vi "ReCalc_V2.00.vi"(3 "Berechnen":bool, 4 "Datenspeicher":T2={"Fahrzeugdaten"="", "date/time string"="", "Rolle [Inkr/U]"=0, "Rollenumfang [m]"=0.0, "Rollenträgheit [kgm²]"=0.0, "Zündung [Imp/U]"=0.0, "Getriebe [1:]"=0.0, "Reifenumfang [m] "=0.0, "element"=0.0, "Gl. Mittelwert"=0, "Differenzenquotient"=0, "Polynom"=0, "dT [s]"=0.0, "element"=0.0, "Lufttemperatur [°C]"=0.0, "Luftfeuchtigkeit [%]"=0.0, "Luftdruck [mbar]"=0.0, [], [], "Best Polynomial Fit"=[], [], "Übersetzung ermitteln aus"=0, "[s]"=0.0, "nmin [1/min]"=0.0, "nmax [1/min]"=0.0, "n vom Gas [1/min]"=0.0, "dT ungefiltert [s]"=[], [], "Boolesch"=FALSE, "Serielle Schnittstelle"="COM4", "nKuWe/nRolle 2"=10.0, "v vom Gas [km/h]"=5000.0}) -> ()   [LabVIEW 2014]
uses:
  <vilib>/Utility/miscctls.llb/LVPointTypeDef.ctl
  <vilib>/Analysis/3filter.llb/IIR Filter (DBL).vi
  <vilib>/Analysis/NI_AALBase.lvlib
panel:
  in  "v vom Gas [km/h]":dbl=5000.0
  in  "Legende":bool=TRUE
  out "Fahrzeugdaten":string
  out "Überlagerung":bool
  in  "Überlagern":bool
  out "Übersetzung ermitteln aus":T1(ring)
  in  "Speichern":bool
  out "Reifenumfang [m]":dbl=1.222
  out "Getriebe [1:]":dbl=5.343
  out "Zündung [Imp/U]":dbl=1.0
  out "Rollengeber [Inkr/U]":u16=200
  out "Luftdruck [mbar]":dbl=1013.0
  out "Luftfeuchtigkeit [%]":dbl=50.0
  out "Lufttemperatur [°C]":dbl=20.0
  in  "Stopp":bool
  in  "Rollenträgheit [kgm²]":dbl=0.402
  in  "Gl. Mittelwert":u8=35
  in  "Differenzenquotient":u8=12
  in  "n vom Gas [1/min]":dbl=5000.0
  out "Rollenumfang [m]":dbl=0.613 format="%.3f"
  out "Datum, Zeit":string
  out "Untersetzung aus:":dbl=2.68 format="%.2f"
  in  "Drucken":bool
  out "Pmax":string
  out "Ergebnis":string
  out "XY-Graph":cluster{dbl[], dbl[]}[](graph)
  in  "Öffnen":bool
  out "korr":dbl
  out "[s]":dbl=5.0
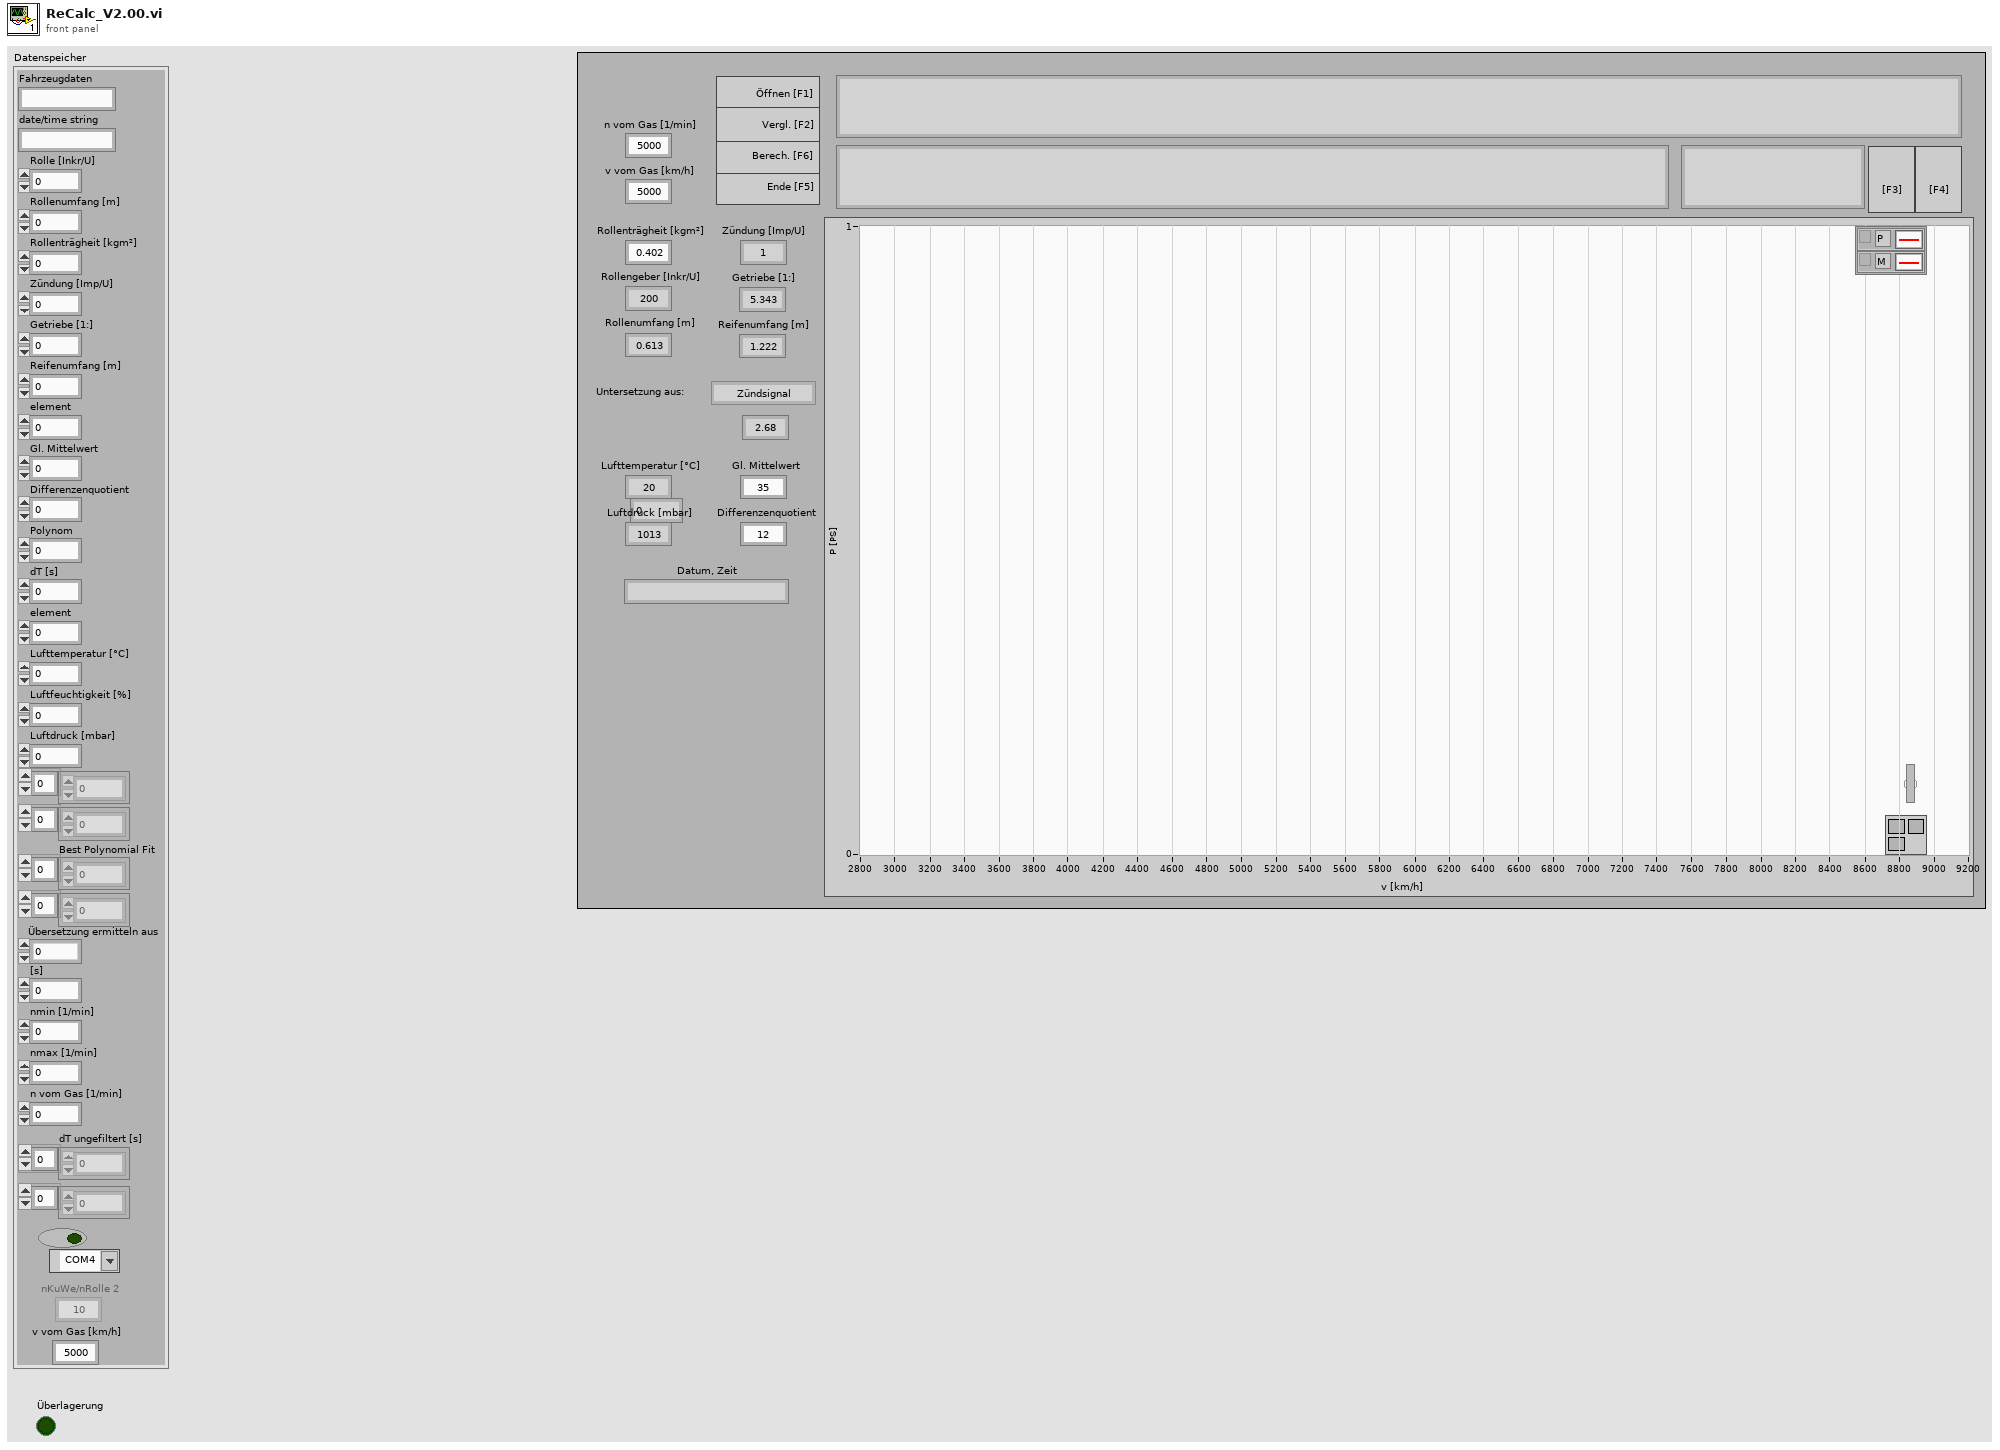
[diagram p1: front panel]
types:
  T1 = enum8{"Zündsignal", "Getriebe & Reifen", "nKuWe / nRolle", "Vario [km/h]"}
  T2 = cluster{"Fahrzeugdaten":string, "date/time string":string, "Rolle [Inkr/U]":u16, "Rollenumfang [m]":dbl, "Rollenträgheit [kgm²]":dbl, "Zündung [Imp/U]":dbl, "Getriebe [1:]":dbl, "Reifenumfang [m] ":dbl, "element":dbl, "Gl. Mittelwert":u8, "Differenzenquotient":u8, "Polynom":u8, "dT [s]":dbl, "element":dbl, "Lufttemperatur [°C]":dbl, "Luftfeuchtigkeit [%]":dbl, "Luftdruck [mbar]":dbl, dbl[], dbl[], "Best Polynomial Fit":dbl[], dbl[], "Übersetzung ermitteln aus":u8, "[s]":dbl, "nmin [1/min]":dbl, "nmax [1/min]":dbl, "n vom Gas [1/min]":dbl, "dT ungefiltert [s]":dbl[], i32[], "Boolesch":bool, "Serielle Schnittstelle":refnum<visa-resource-name>, "nKuWe/nRolle 2":dbl, "v vom Gas [km/h]":dbl}
  T3 = typedef "LVPointTypeDef.ctl" = cluster{"Horizontal":i16, "Vertical":i16}
  T4 = enum16{"Zündsignal", "Getriebe & Reifen", "nKuWe / nRolle", "Vario (km/h)"}
  T5 = cluster{"Fahrzeugdaten":string, "date/time string":string, "Rolle [Inkr/U]":u16, "Rollenumfang [m]":dbl, "Rollenträgheit [kgm²]":dbl, "Zündung [Imp/U]":dbl, "Getriebe [1:]":dbl, "Reifenumfang [m] ":dbl, "element":dbl, "Gl. Mittelwert":u8, "Differenzenquotient":u8, "Polynom":u8, "dT [s]":dbl, "element":dbl, "Lufttemperatur [°C]":dbl, "Luftfeuchtigkeit [%]":dbl, "Luftdruck [mbar]":dbl, dbl[], dbl[], "Best Polynomial Fit":dbl[], dbl[], "Übersetzung ermitteln aus":u8, "[s]":dbl, "nmin [1/min]":dbl, "nmax [1/min]":dbl, "n vom Gas [1/min]":dbl, "dT-Array [s]":dbl[], i32[], "Boolesch":bool, "Serielle Schnittstelle":refnum<visa-resource-name>, "nKuWe/nRolle":dbl, "v vom Gas [km/h]":dbl}
  T6 = enum8{"Enabled", "Disabled", "Disabled and Grayed Out"}
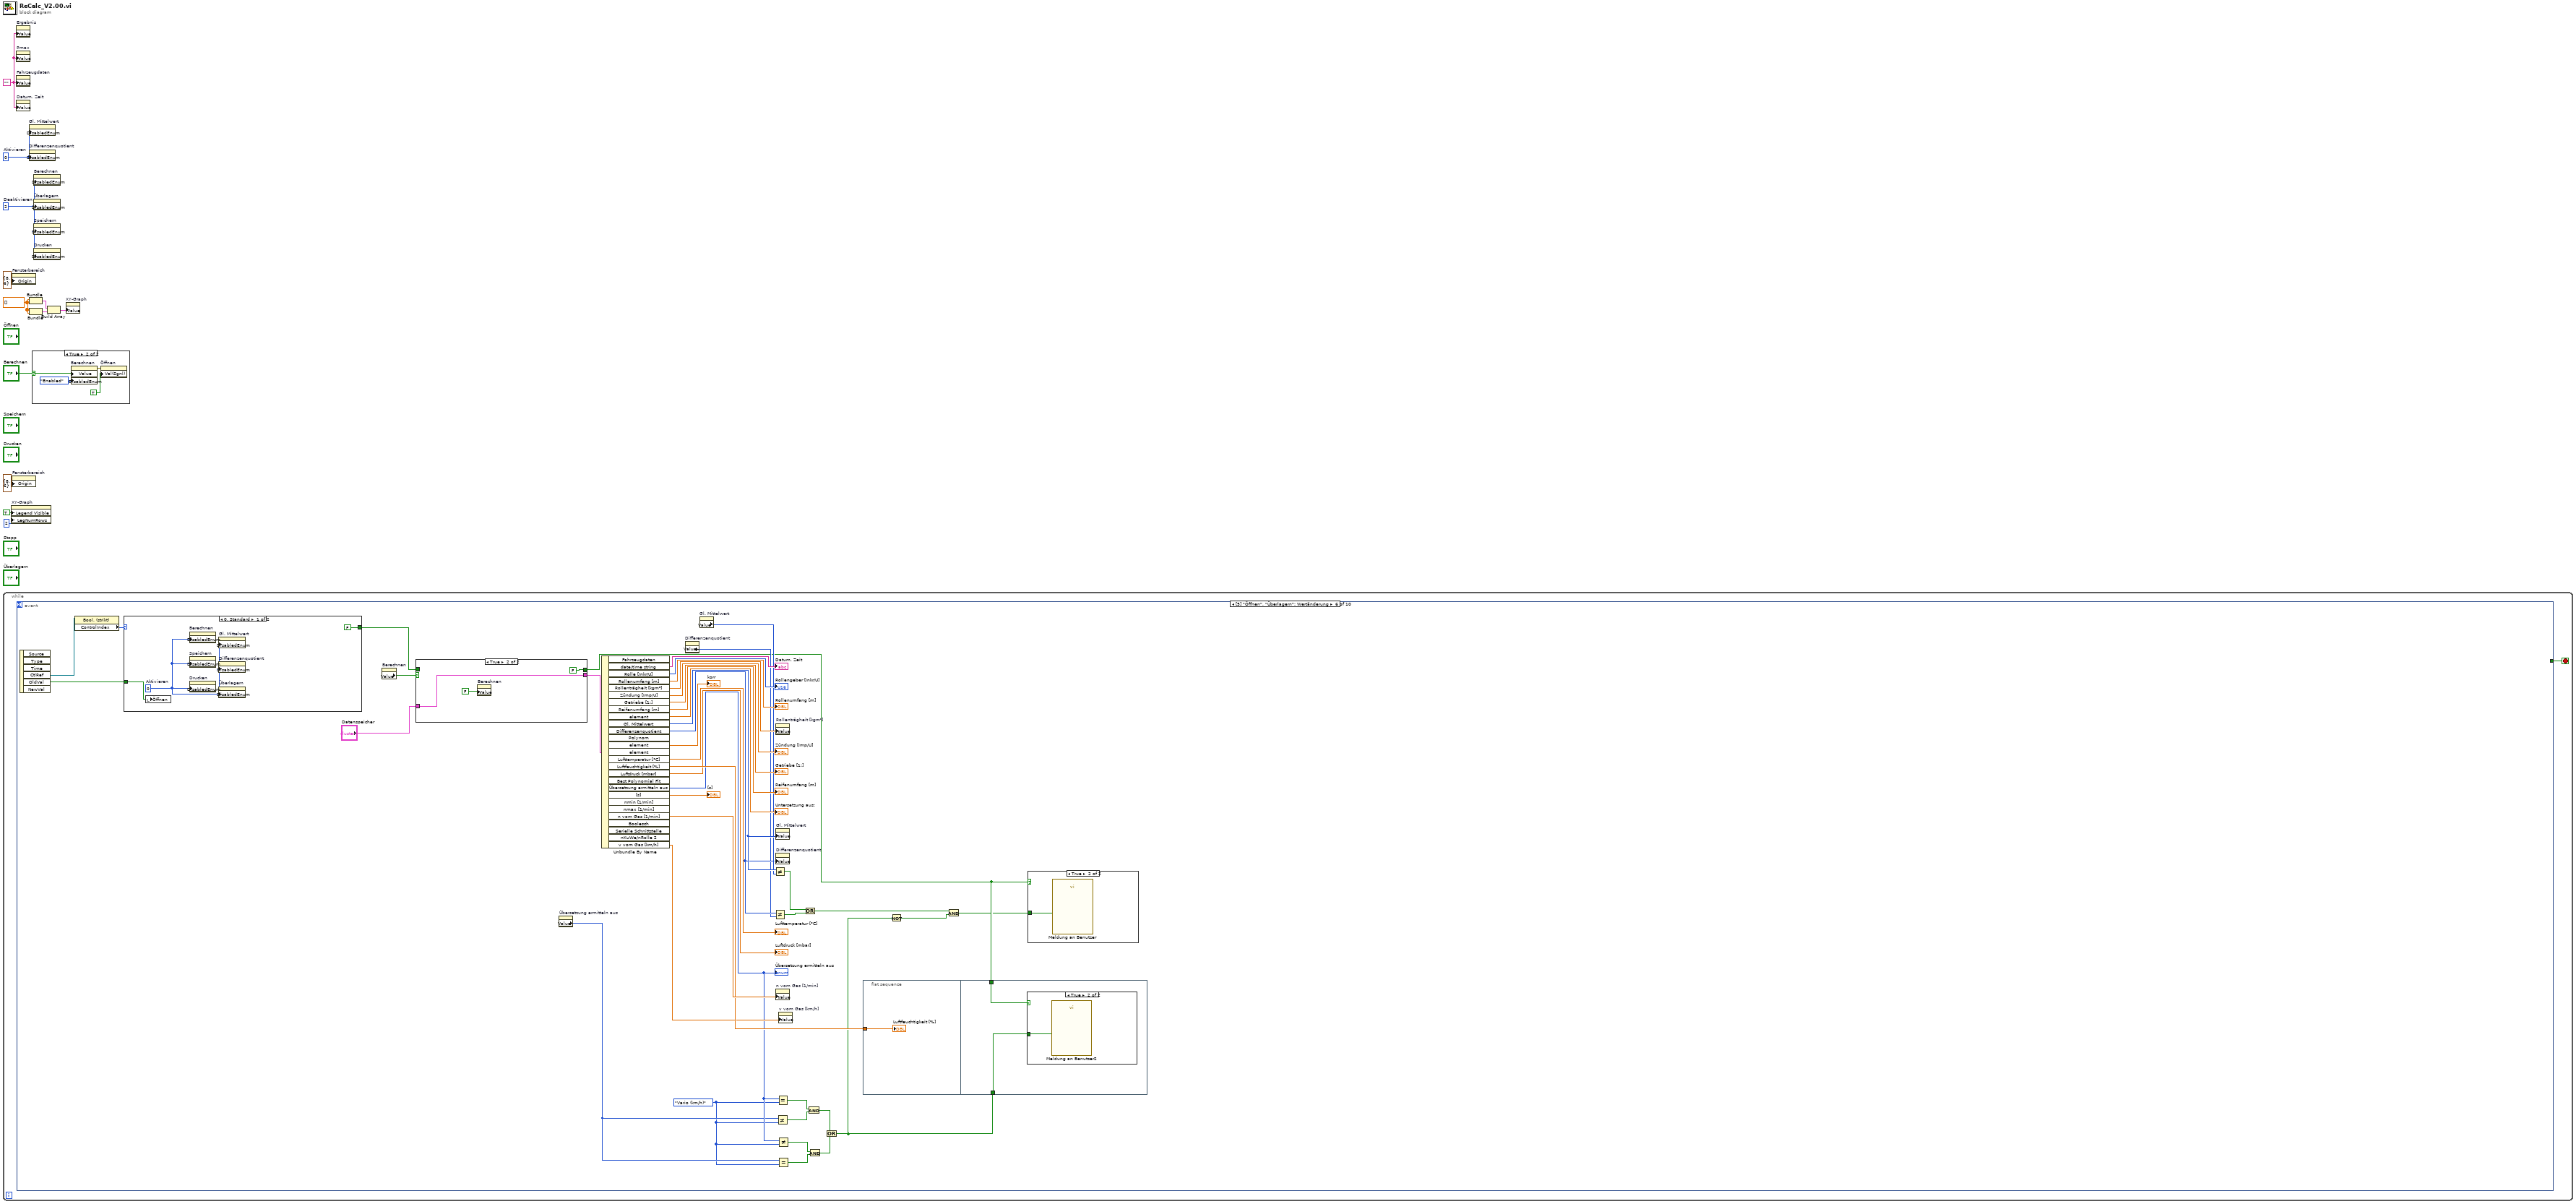
[diagram p0: block diagram]
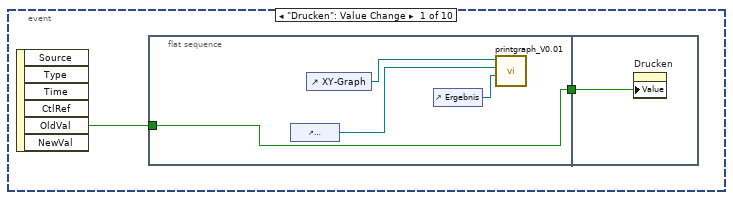
[diagram p3: hidden frame]
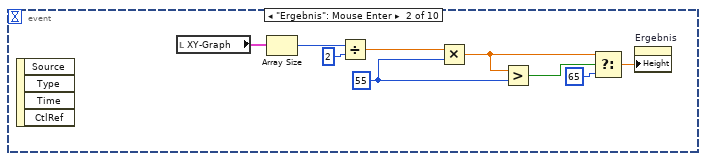
[diagram p4: hidden frame]
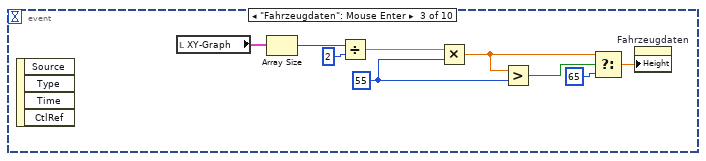
[diagram p5: hidden frame]
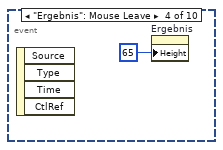
[diagram p6: hidden frame]
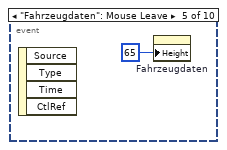
[diagram p7: hidden frame]
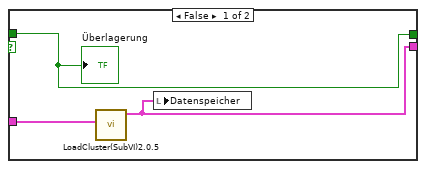
[diagram p9: hidden frame]
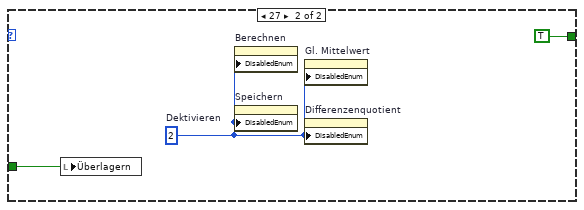
[diagram p11: hidden frame]
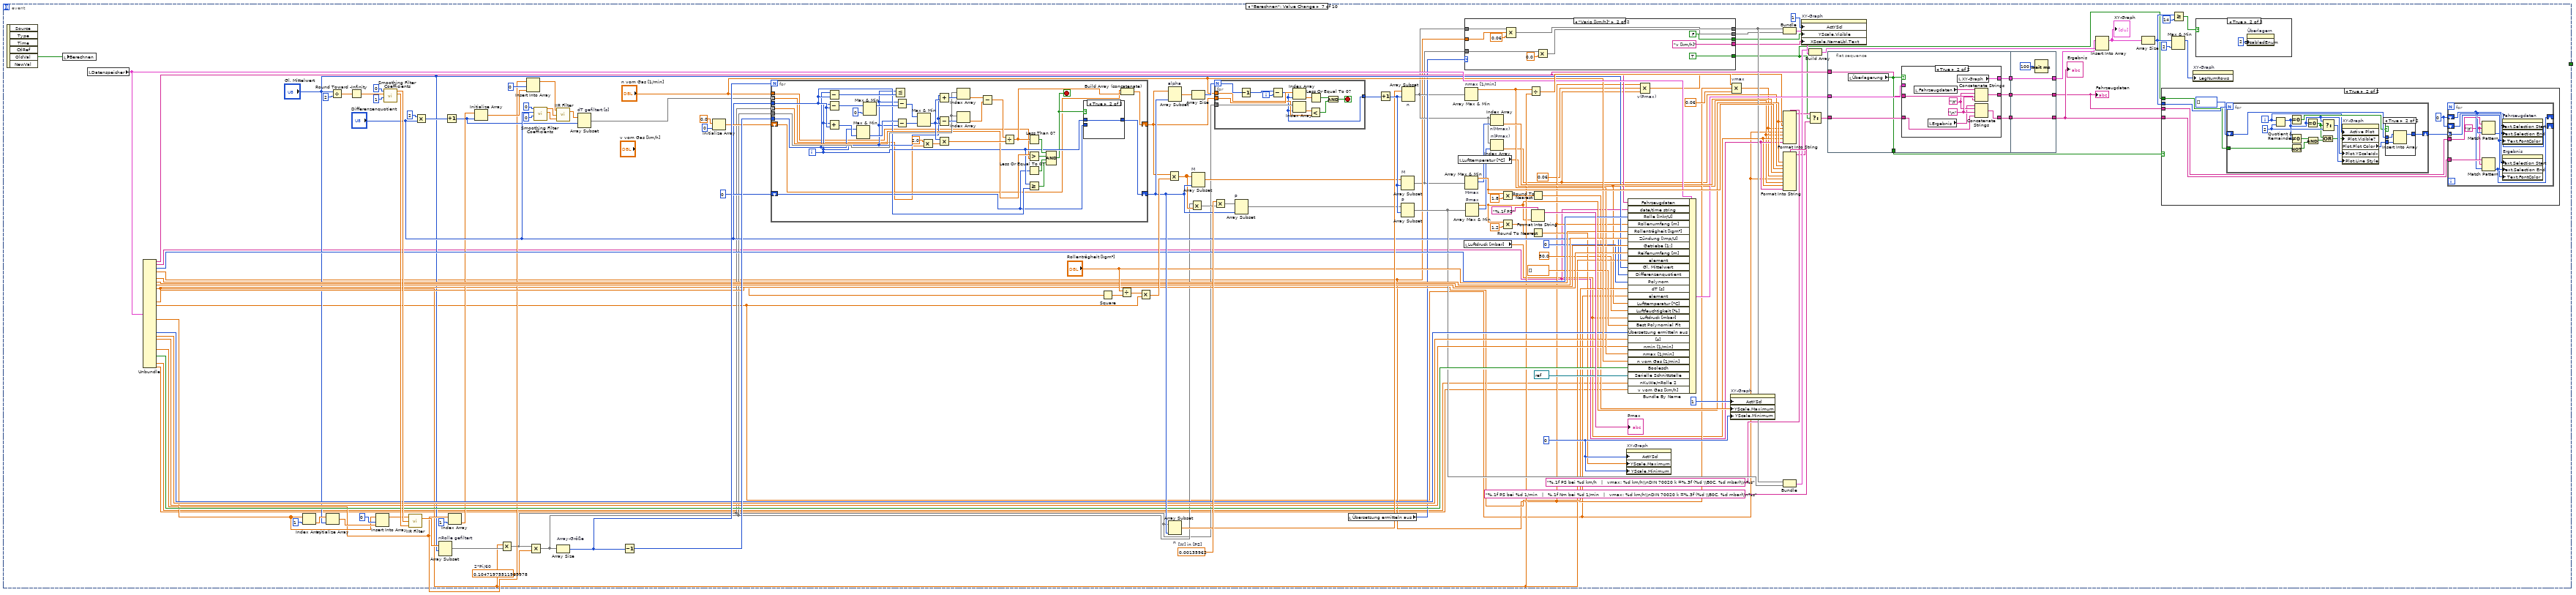
[diagram p12: hidden frame]
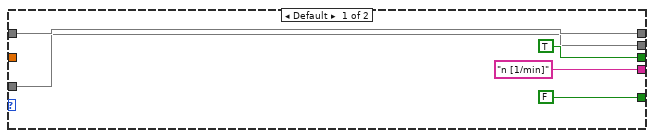
[diagram p13: hidden frame]
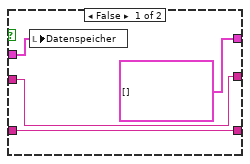
[diagram p15: hidden frame]
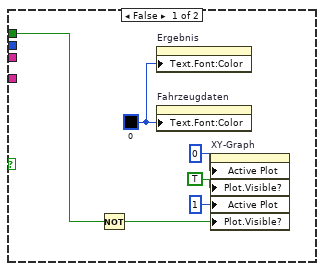
[diagram p16: hidden frame]
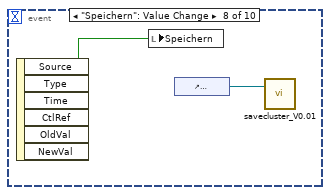
[diagram p19: hidden frame]
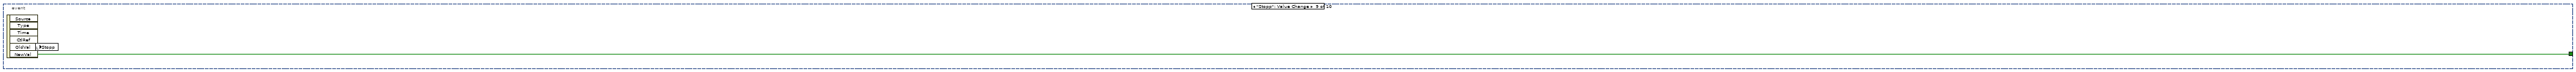
[diagram p20: hidden frame]
diagram:
  w2 = 0  # Aktivieren
  w8 = dbl[] []
  w4 = 2  # Deaktivieren
  w12 = ""
  n1 = while {
    stop <- w13 stop-if-true
    n2 = event shown="[5] \"Öffnen\", \"Überlagern\": Wertänderung" {
      selector: _ -> [_ _ _ _ _ _ _ _ _ _]
      dyn-events: _ -> [_ _ _ _ _ _ _ _ _ _]
      timeout: _ -> [_ _ _ _ _ _ _ _ _ _]
      tunnel: [_ _ _ _ _ _ _ _ w367 _] -> w13
      event "Drucken": Value Change {
        n3 = event-data() -> ("OldVal"=w15:bool)  [unwired: 1 in, 5 out]
        n4 = flat-sequence {
          tunnel: w15 -> [w19]
          tunnel: [w19] -> w14
          tunnel: w14 -> [w20]
          frame #0 {
            n5 = control-ref of="Fahrzeugdaten"() -> (w17:refnum<vi>)
            n6 = control-ref of="XY-Graph"() -> (w18:refnum<vi>)
            n7 = control-ref of="Ergebnis"() -> (w16:refnum<vi>)
            n8 = call "printgraph_V0.01.vi"("reference 2"=w16, "Fahrzeugdaten"=w17, "XYGraph (Eingang)"=w18) -> ()  [unwired: 9 in]
          }
          frame #1 {
            n9 = property on="Drucken" class="Bool. (strikt)"("Value"=w20) -> ()  [unwired: 2 in, 2 out]
          }
        }
      }
      event "Ergebnis": Mouse Enter {
        w23 = u32 55 ("Größe:Höhe")
        n10 = event-data() -> ()  [unwired: 1 in, 4 out]
        n11 = local read "XY-Graph"() -> (w29:cluster{dbl[], dbl[]}[])
        n12 = Array Size(array=w29) -> (size(s)=w28:i32)
        n13 = Divide(x=w28, y=2) -> (x/y=w26:dbl)
        n14 = Multiply(x=w26, y=w23) -> (x*y=w24:dbl)
        n15 = Greater?(x=w24, y=w23) -> (0:w25:bool)
        n16 = Select(t=w24, s=w25, f=u32 65 ("Größe:Höhe")) -> (s? t:f=w22:dbl)
        n17 = property on="Ergebnis" class="Str"("Height"=w22) -> ()  [unwired: 2 in, 2 out]
      }
      event "Fahrzeugdaten": Mouse Enter {
        w32 = u32 55 ("Größe:Höhe")
        n18 = event-data() -> ()  [unwired: 1 in, 4 out]
        n19 = local read "XY-Graph"() -> (w38:cluster{dbl[], dbl[]}[])
        n20 = Array Size(array=w38) -> (size(s)=w37:i32)
        n21 = Divide(x=w37, y=2) -> (x/y=w35:dbl)
        n22 = Multiply(x=w35, y=w32) -> (x*y=w33:dbl)
        n23 = Greater?(x=w33, y=w32) -> (0:w34:bool)
        n24 = Select(t=w33, s=w34, f=u32 65 ("Größe:Höhe")) -> (s? t:f=w31:dbl)
        n25 = property on="Fahrzeugdaten" class="Str"("Height"=w31) -> ()  [unwired: 2 in, 2 out]
      }
      event "Ergebnis": Mouse Leave {
        n26 = event-data() -> ()  [unwired: 1 in, 4 out]
        n27 = property on="Ergebnis" class="Str"("Height"=u32 65 ("Größe:Höhe")) -> ()  [unwired: 2 in, 2 out]
      }
      event "Fahrzeugdaten": Mouse Leave {
        n28 = event-data() -> ()  [unwired: 1 in, 4 out]
        n29 = property on="Fahrzeugdaten" class="Str"("Height"=u32 65 ("Größe:Höhe")) -> ()  [unwired: 2 in, 2 out]
      }
      event "Öffnen", "Überlagern": Value Change {
        w50 = T4."Vario (km/h)"
        n30 = event-data() -> ("CtlRef"=w81:refnum<vi>, "OldVal"=w79:bool)  [unwired: 1 in, 4 out]
        n31 = property class="Bool. (strikt)"(reference=w81) -> ("ControlIndex"=w80:i32)  [unwired: 1 in, 2 out]
        n32 = case shown="0, Standard" w80 {
          tunnel: w79 -> [w96 w99]
          tunnel: [FALSE ("Überlagerung") TRUE ("Überlagerung")] -> w78
          frame 0, Default {
            w94 = 0  # Aktivieren
            n33 = local write "Öffnen"(w96) -> ()
            n34 = property on="Berechnen" class="Bool. (strikt)"("DisabledEnum"=w94) -> ()  [unwired: 2 in, 2 out]
            n35 = property on="Speichern" class="Bool. (strikt)"("DisabledEnum"=w94) -> ()  [unwired: 2 in, 2 out]
            n36 = property on="Drucken" class="Bool. (strikt)"("DisabledEnum"=w94) -> ()  [unwired: 2 in, 2 out]
            n37 = property on="Gl. Mittelwert" class="DigWert (strikt)"("DisabledEnum"=w94) -> ()  [unwired: 2 in, 2 out]
            n38 = property on="Differenzenquotient" class="DigWert (strikt)"("DisabledEnum"=w94) -> ()  [unwired: 2 in, 2 out]
            n39 = property on="Überlagern" class="Bool. (strikt)"("DisabledEnum"=w94) -> ()  [unwired: 2 in, 2 out]
          }
          frame 27 {
            w97 = 2  # Dektivieren
            n40 = local write "Überlagern"(w99) -> ()
            n41 = property on="Berechnen" class="Bool. (strikt)"("DisabledEnum"=w97) -> ()  [unwired: 2 in, 2 out]
            n42 = property on="Speichern" class="Bool. (strikt)"("DisabledEnum"=w97) -> ()  [unwired: 2 in, 2 out]
            n43 = property on="Gl. Mittelwert" class="DigWert (strikt)"("DisabledEnum"=w97) -> ()  [unwired: 2 in, 2 out]
            n44 = property on="Differenzenquotient" class="DigWert (strikt)"("DisabledEnum"=w97) -> ()  [unwired: 2 in, 2 out]
          }
        }
        n45 = property on="Berechnen" class="Bool. (strikt)"() -> ("Value"=w63:bool)  [unwired: 2 in, 2 out]
        n46 = case shown="True" w63 {
          tunnel: "Datenspeicher" -> [w85 w88]
          tunnel: w78 -> [w86 _]
          tunnel: [w84 w88] -> w64
          tunnel: [w86 FALSE] -> w45
          frame False {
            n47 = call "LoadCluster(SubVI)2.0.5.vi"("Datenspeicher"=w85) -> ("Value"=w84:T5)  [unwired: 10 in]
            n48 = local write "Datenspeicher"(w84) -> ()
            "Überlagerung" <- w86
          }
          frame True {
            n49 = property on="Berechnen" class="Bool. (strikt)"("Value"=FALSE) -> ()  [unwired: 2 in, 2 out]
          }
        }
        n50 = property on="Übersetzung ermitteln aus" class="Enum (strikt)"() -> ("Value"=w51:T1)  [unwired: 2 in, 2 out]
        n51 = Unbundle By Name(w64) -> ("date/time string"=→"Datum, Zeit":string, "Rolle [Inkr/U]"=→"Rollengeber [Inkr/U]":u16, "Rollenumfang [m]"=→"Rollenumfang [m]":dbl, "Rollenträgheit [kgm²]"=w68:dbl, "Zündung [Imp/U]"=→"Zündung [Imp/U]":dbl, "Getriebe [1:]"=→"Getriebe [1:]":dbl, "Reifenumfang [m]"=→"Reifenumfang [m]":dbl, "element"=→"Untersetzung aus:":dbl, "Gl. Mittelwert"=w62:u8, "Differenzenquotient"=w60:u8, "element"=→"korr":dbl, "Lufttemperatur [°C]"=→"Lufttemperatur [°C]":dbl, "Luftfeuchtigkeit [%]"=w75:dbl, "Luftdruck [mbar]"=→"Luftdruck [mbar]":dbl, "Übersetzung ermitteln aus"=w52:u8, "[s]"=→"[s]":dbl, "n vom Gas [1/min]"=w77:dbl, "v vom Gas [km/h]"=w55:dbl)  [unwired: 9 out]
        "Übersetzung ermitteln aus" <- w52
        n52 = property on="Differenzenquotient" class="DigWert (strikt)"() -> ("Value"=w59:u8)  [unwired: 2 in, 2 out]
        n53 = property on="Gl. Mittelwert" class="DigWert (strikt)"() -> ("Value"=w61:u8)  [unwired: 2 in, 2 out]
        n54 = Not Equal?(x=w62, y=w61) -> (x != y?=w58:bool)
        n55 = Not Equal?(x=w60, y=w59) -> (x != y?=w57:bool)
        n56 = property on="Rollenträgheit [kgm²]" class="DigWert (strikt)"("Value"=w68) -> ()  [unwired: 2 in, 2 out]
        n57 = property on="Gl. Mittelwert" class="DigWert (strikt)"("Value"=w62) -> ()  [unwired: 2 in, 2 out]
        n58 = property on="Differenzenquotient" class="DigWert (strikt)"("Value"=w60) -> ()  [unwired: 2 in, 2 out]
        n59 = property on="n vom Gas [1/min]" class="DigWert (strikt)"("Value"=w77) -> ()  [unwired: 2 in, 2 out]
        n60 = Not Equal?(x=w51, y=w50) -> (x != y?=w53:bool)
        n61 = Equal?(x=w52, y=w50) -> (x = y?=w54:bool)
        n62 = Not Equal?(x=w52, y=w50) -> (x != y?=w49:bool)
        n63 = Equal?(x=w51, y=w50) -> (x = y?=w48:bool)
        n64 = property on="v vom Gas [km/h]" class="DigWert (strikt)"("Value"=w55) -> ()  [unwired: 2 in, 2 out]
        n65 = Or(x=w58, y=w57) -> (x .or. y?=w41:bool)
        n66 = And(x=w54, y=w53) -> (x .and. y?=w47:bool)
        n67 = And(x=w49, y=w48) -> (x .and. y?=w46:bool)
        n68 = Or(x=w47, y=w46) -> (x .or. y?=w43:bool)
        n69 = flat-sequence {
          tunnel: w75 -> [w90]
          tunnel: w45 -> [w92]
          tunnel: w43 -> [w91]
          frame #0 {
            "Luftfeuchtigkeit [%]" <- w90
          }
          frame #1 {
            n70 = case shown="True" w92 {
              tunnel: w91 -> [_ w93]
              frame False {
              }
              frame True {
                n71 = call "Meldung an Benutzer2"("Enable"=w93) -> ()  [unwired: 9 in, 2 out]
              }
            }
          }
        }
        n72 = Not(x=w43) -> (.not. x?=w42:bool)
        n73 = And(x=w41, y=w42) -> (x .and. y?=w44:bool)
        n74 = case shown="True" w45 {
          tunnel: w44 -> [_ w83]
          frame False {
          }
          frame True {
            n75 = call "Meldung an Benutzer"("Enable"=w83) -> ()  [unwired: 9 in, 2 out]
          }
        }
      }
      event "Berechnen": Value Change {
        w210 = 0
        w224 = 0.00135962  # [W] in [PS]
        w231 = 0.10471975511965978  # 2*Pi/60
        n76 = event-data() -> ("OldVal"=w180:bool)  [unwired: 1 in, 5 out]
        n77 = local write "Berechnen"(w180) -> ()
        n78 = local read "Datenspeicher"() -> (w193:T2)
        n79 = Unbundle(w193) -> ("Fahrzeugdaten"=w172:string, "date/time string"=w115:string, "Rolle [Inkr/U]"=w192:u16, "Rollenumfang [m]"=w118:dbl, "Zündung [Imp/U]"=w186:dbl, "Getriebe [1:]"=w185:dbl, "Reifenumfang [m]"=w184:dbl, "element"=w134:dbl, "dT [s]"=w144:dbl, "element"=w112:dbl, w143:dbl[], "Übersetzung ermitteln aus"=w187:u8, "[s]"=w181:dbl, "nmin [1/min]"=w182:dbl, "dT ungefiltert [s]"=w142:dbl[], "Boolesch"=w189:bool, "nKuWe/nRolle 2"=w100:dbl, "v vom Gas [km/h]"=w101:dbl)  [unwired: 14 out]
        n80 = Index Array(array=w143, index=1) -> (element=w198:dbl)
        n81 = Initialize Array(w198, "Gl. Mittelwert") -> (w199:dbl[])
        n82 = Divide(x="Gl. Mittelwert", y=2) -> (x/y=w234:dbl)
        n83 = Round Toward -Infinity(1:w234) -> (0:w233:dbl)
        n84 = Insert Into Array ("In Array einfügen")(array=w143, index=0, new element=w199) -> (w196:dbl[])
        n85 = call <vilib>:"Smoothing Filter Coefficients.vi"("shape"=1, "half-width"=w233, "type"=0) -> ("forward coefficients"=w200:dbl[], "reverse coefficients"=w201:dbl[])  [unwired: 6 in, 1 out]
        n86 = call-poly <vilib>:"IIR Filter.vi"("Forward Coefficients"=w200, "Reverse Coefficients"=w201, "X"=w196) -> ("Filtered X"=w195:dbl[])  [unwired: 1 in, 1 out]
        n87 = Multiply(x=2, y="Differenzenquotient") -> (x*y=w152:i32)
        n88 = Array Subset "nRolle gefiltert"(array=w195, index="Gl. Mittelwert") -> (w136:dbl[])  [unwired: 1 in]
        n89 = Increment(x=w152) -> (x+1=w145:i32)
        n90 = Index Array(array=w142, index=1 ("Index")) -> (element=w150:dbl)
        n91 = Initialize Array(w150, w145) -> (w148:dbl[])
        n92 = Multiply(x=w134, y=w136) -> (x*y=w135:dbl[])
        n93 = Insert Into Array(array=w142, index=0 ("Index"), new element=w148) -> (w147:dbl[])
        n94 = Multiply(x=w135, y=w231) -> (x*y=w138:dbl[])
        n95 = call <vilib>:"Smoothing Filter Coefficients.vi"("shape"=0, "half-width"="Differenzenquotient", "type"=0) -> ("forward coefficients"=w155:dbl[], "reverse coefficients"=w156:dbl[])  [unwired: 6 in, 1 out]
        n96 = call-poly <vilib>:"IIR Filter.vi"("Forward Coefficients"=w155, "Reverse Coefficients"=w156, "X"=w147) -> ("Filtered X"=w146:dbl[])  [unwired: 1 in, 1 out]
        n97 = Array Size "Array-Größe"(array=w138) -> (size(s)=w229:i32)
        n98 = Array Subset "dT gefiltert [s]"(array=w146, index=w145) -> (w137:dbl[])  [unwired: 1 in]
        n99 = Decrement(x=w229) -> (x-1=w230:i32)
        n100 = Initialize Array(0.0 ("y"), 0) -> (w226:dbl[])
        n101 = for {
          N: w229 -> [_]
          tunnel: "Differenzenquotient" -> [w342]
          tunnel: w138 -> [w348]
          tunnel: w230 -> [w341]
          shift-right: [w346] -> w139
          shift-left: w226 -> [w329]
          tunnel: w135 -> [w344] mode=indexing
          tunnel: "n vom Gas [1/min]" -> [w333]
          shift-right: [w332] -> w217
          shift-left: 0 -> [w335]
          tunnel: w137 -> [w328] mode=indexing
          i -> [w336]
          stop <- w334 stop-if-true
          n102 = Subtract(x=w341, y=w342) -> (x-y=w343:i32)
          n103 = Subtract(x=w336, y=w342) -> (x-y=w361:i32)
          n104 = Add(x=w336, y=w342) -> (x+y=w355:i32)
          n105 = Max & Min(x=w341, y=w355) -> (min(x,y)=w356:i32)  [unwired: 1 out]
          n106 = Max & Min(x=w361, y=0) -> (max(x,y)=w359:i32)  [unwired: 1 out]
          n107 = Less Or Equal?(x=w336, y=w343) -> ()  [unwired: 1 out]
          n108 = Subtract(x=w336, y=w359) -> (x-y=w358:i32)
          n109 = Subtract(x=w356, y=w336) -> (x-y=w357:i32)
          n110 = Max & Min(x=w358, y=w357) -> (min(x,y)=w349:i32)  [unwired: 1 out]
          n111 = Multiply(x=2.0, y=w328) -> (x*y=w330:dbl)
          n112 = Add(x=w336, y=w349) -> (x+y=w354:i32)
          n113 = Subtract(x=w336, y=w349) -> (x-y=w353:i32)
          n114 = Multiply(x=w349, y=w330) -> (x*y=w347:dbl)
          n115 = Index Array(array=w348, index=w354) -> (element=w351:dbl)
          n116 = Index Array(array=w348, index=w353) -> (element=w352:dbl)
          n117 = Subtract(x=w351, y=w352) -> (x-y=w350:dbl)
          n118 = Divide(x=w350, y=w347) -> (x/y=w340:dbl)
          n119 = Less Than 0?(x=w340) -> (x < 0?=w338:bool)
          n120 = Greater?(x=w344, y=w333) -> (0:w345:bool)
          n121 = Less Or Equal To 0?(x=w335) -> (x <= 0?=w337:bool)
          n122 = Greater Or Equal?(x=w336, y=w342) -> (x >= y?=w339:bool)
          n123 = Compound Arithmetic op=AND(w338, w345, w337, w339) -> (w334:bool)
          n124 = case shown="True" w334 {
            tunnel: w336 -> [_ w363]
            tunnel: [w362 w363] -> w332
            tunnel: w335 -> [w362 _]
            frame False {
            }
            frame True {
            }
          }
          n125 = Build Array (concatenate)(w329, w340) -> (w346:dbl[])
        }
        n126 = Square(x=w134) -> (x^2=w225:dbl)
        n127 = Divide(x="Rollenträgheit [kgm²]", y=w225) -> (x/y=w222:dbl)
        n128 = Multiply(x=w222, y=w112) -> (x*y=w221:dbl)
        n129 = Multiply(x=w139, y=w221) -> (x*y=w204:dbl[])
        n130 = Array Subset "alpha"(array=w139, length=w217) -> (w219:dbl[])  [unwired: 1 in]
        n131 = Array Subset "n"(array=w135, length=w217) -> (w202:dbl[])  [unwired: 1 in]
        n132 = Multiply(x=w138, y=w204) -> (x*y=w223:dbl[])
        n133 = Array Size(array=w219) -> (size(s)=w216:i32)
        n134 = Array Subset "M"(array=w204, length=w217) -> (w141:dbl[])  [unwired: 1 in]
        n135 = Multiply(x=w224, y=w223) -> (x*y=w218:dbl[])
        n136 = for {
          N: w216 -> [w327]
          tunnel: w139 -> [w324]
          tunnel: w135 -> [w321]
          tunnel: "n vom Gas [1/min]" -> [w318]
          tunnel: [w316] -> w215
          i -> [w322]
          stop <- w317 stop-if-true
          n137 = Decrement(x=w327) -> (x-1=w326:i32)
          n138 = Subtract(x=w326, y=w322) -> (x-y=w316:i32)
          n139 = Index Array(array=w324, index=w316) -> (element=w325:dbl)
          n140 = Index Array(array=w321, index=w316) -> (element=w320:dbl)
          n141 = Less?(x=w320, y=w318) -> (x < y?=w319:bool)
          n142 = Less Or Equal To 0?(x=w325) -> (x <= 0?=w323:bool)
          n143 = And(x=w323, y=w319) -> (x .and. y?=w317:bool)
        }
        n144 = Array Subset "P"(array=w218, length=w217) -> (w140:dbl[])  [unwired: 1 in]
        n145 = local read "Übersetzung ermitteln aus"() -> (w124:T1)
        n146 = Increment(x=w215) -> (x+1=w214:i32)
        n147 = Array Subset "M"(array=w141, index=w214) -> (w103:dbl[])  [unwired: 1 in]
        n148 = Array Subset "P"(array=w140, index=w214) -> (w164:dbl[])  [unwired: 1 in]
        n149 = Array Subset "n"(array=w202, index=w214) -> (w123:dbl[])  [unwired: 1 in]
        n150 = local read "Lufttemperatur [°C]"() -> (w113:dbl)
        n151 = local read "Luftdruck [mbar]"() -> (w114:dbl)
        n152 = case shown="\"Vario [km/h]\"" w124 {
          tunnel: w118 -> [_ w250]
          tunnel: w123 -> [w241 w249]
          tunnel: [w241 w248] -> w122
          tunnel: [FALSE TRUE] -> w104
          tunnel: [TRUE FALSE] -> w106
          tunnel: ["n [1/min]" "v [km/h]"] -> w105
          tunnel: w103 -> [w237 w243]
          tunnel: [w237 w244] -> w102
          frame Default {
          }
          frame "Vario [km/h]" {
            n153 = Compound Arithmetic op=MULTIPLY(w249, w250, 0.06) -> (w248:dbl[])
            n154 = Multiply(x=w243, y=0.0) -> (x*y=w244:dbl[])
          }
        }
        n155 = Array Max & Min "nmax [1/min]"(array=w123) -> (max value=w183:dbl)  [unwired: 3 out]
        n156 = Array Max & Min "Mmax"(array=w103) -> (max value=w206:dbl, max index (indices)=w162:i32)  [unwired: 2 out]
        n157 = Array Max & Min "Pmax"(array=w164) -> (max value=w120:dbl, max index (indices)=w161:i32)  [unwired: 2 out]
        n158 = Index Array "n(Mmax)"(array=w123, index=w162) -> (element=w188:dbl)
        n159 = Index Array "n(Pmax)"(array=w123, index=w161) -> (element=w116:dbl)
        n160 = Multiply(x=w206, y=1.8) -> (x*y=w133:dbl)
        n161 = Multiply(x=w120, y=1.2) -> (x*y=w130:dbl)
        n162 = Divide(x=w183, y=w134) -> (x/y=w209:dbl)
        n163 = Format Into String(format string="%.1f PS" ("Format-String"), w120) -> (resulting string=→"Pmax":string)  [unwired: 2 in, 1 out]
        n164 = Round To Nearest(number=w133) -> (nearest integer value=w132:dbl)
        n165 = Round To Nearest(number=w130) -> (nearest integer value=w131:dbl)
        n166 = property on="XY-Graph" class="XYGraph (strikt)"("ActYScl"=w210, "YScale.Maximum"=w131, "YScale.Minimum"=w210) -> ()  [unwired: 2 in, 2 out]
        n167 = Bundle By Name(cluster=w193, "Fahrzeugdaten"=w172, "date/time string"=w115, "Rolle [Inkr/U]"=w192, "Rollenumfang [m]"=w118, "Rollenträgheit [kgm²]"="Rollenträgheit [kgm²]", "Zündung [Imp/U]"=w186, "Getriebe [1:]"=w185, "Reifenumfang [m]"=w184, "element"=w134, "Gl. Mittelwert"="Gl. Mittelwert", "Differenzenquotient"="Differenzenquotient", "Polynom"=0, "dT [s]"=w144, "element"=w112, "Lufttemperatur [°C]"=w113, "Luftfeuchtigkeit [%]"=50.0, "Luftdruck [mbar]"=w114, "Best Polynomial Fit"=dbl[] [], "Übersetzung ermitteln aus"=w187, "[s]"=w181, "nmin [1/min]"=w182, "nmax [1/min]"=w183, "n vom Gas [1/min]"="n vom Gas [1/min]", "Boolesch"=w189, "Serielle Schnittstelle"=refnum<visa-resource-name> refnum, "nKuWe/nRolle 2"=w100, "v vom Gas [km/h]"=w101) -> (w178:T2)
        n168 = Compound Arithmetic op=MULTIPLY "v(Pmax)"(w118, 0.06, w116) -> (w119:dbl)
        n169 = property on="XY-Graph" class="XYGraph (strikt)"("ActYScl"=1, "YScale.Maximum"=w132, "YScale.Minimum"=w210) -> ()  [unwired: 2 in, 2 out]
        n170 = Compound Arithmetic op=MULTIPLY "vmax"(w209, w118, 0.06) -> (w111:dbl)
        n171 = Bundle(w122, w102) -> (w166:cluster{dbl[], dbl[]})  [unwired: 1 in]
        n172 = Format Into String(format string="%.1f PS bei %d km/h   |   vmax: %d km/h\\nDIN 70020 k =%.3f (%d \\B0C, %d mbar)\\n%s" ("Format-String"), w120, w119, w111, w112, w113, w114, w115) -> (resulting string=w108:string)  [unwired: 2 in, 1 out]
        n173 = Format Into String(format string="%.1f PS bei %d 1/min   |   %.1f Nm bei %d 1/min   |   vmax: %d km/h\\nDIN 70020 k =%.3f (%d \\B0C, %d mbar)\\n%s" ("Format-String"), w120, w116, w206, w188, w111, w112, w113, w114, w115) -> (resulting string=w109:string)  [unwired: 2 in, 1 out]
        n174 = Bundle(w122, w164) -> (w167:cluster{dbl[], dbl[]})  [unwired: 1 in]
        n175 = property on="XY-Graph" class="XYGraph (strikt)"("ActYScl"=1, "YScale.Visible"=w106, "XScale.NameLbl.Text"=w105) -> ()  [unwired: 2 in, 2 out]
        n176 = Build Array(w167, w166) -> (w176:cluster{dbl[], dbl[]}[])
        n177 = Select(t=w108, s=w104, f=w109) -> (s? t:f=w110:string)
        n178 = flat-sequence {
          tunnel: w110 -> [w259]
          tunnel: w178 -> [w258]
          tunnel: [w257] -> w177
          tunnel: w172 -> [w253]
          tunnel: [w256] -> w171
          tunnel: [w255] -> w170
          tunnel: [w254] -> w169
          tunnel: [w274] -> w173
          tunnel: [w275] -> w174
          tunnel: [w276] -> w175
          tunnel: w171 -> [w276]
          tunnel: w170 -> [w275]
          tunnel: w169 -> [w274]
          frame #0 {
            n179 = local read "Überlagerung"() -> (w257:bool)
            n180 = case shown="True" w257 {
              tunnel: [cluster{dbl[], dbl[]}[] [] ("XY-Graph") w272] -> w256
              tunnel: w259 -> [w262 w270]
              tunnel: [w262 w271] -> w255
              tunnel: w258 -> [w261 _]
              tunnel: w253 -> [w260 w268]
              tunnel: [w260 w267] -> w254
              frame False {
                n181 = local write "Datenspeicher"(w261) -> ()
              }
              frame True {
                w266 = "\t"
                w269 = "\n"
                n182 = local read "Fahrzeugdaten"() -> (w265:string)
                n183 = local read "Ergebnis"() -> (w264:string)
                n184 = local read "XY-Graph"() -> (w272:cluster{dbl[], dbl[]}[])
                n185 = Concatenate Strings(w265, w266, w269, w268) -> (w267:string)
                n186 = Concatenate Strings(w264, w266, w269, w270) -> (w271:string)
              }
            }
          }
          frame #1 {
            n187 = Wait (ms)(milliseconds to wait=u32 100 ("Zu wartende ms")) -> ()  [unwired: 1 out]
          }
        }
        n188 = Insert Into Array(array=w175, new element=w176) -> (w179:cluster{dbl[], dbl[]}[])  [unwired: 1 in]
        "XY-Graph" <- w179
        n189 = Array Size(array=w179) -> (size(s)=w127:i32)
        n190 = case shown="True" w177 {
          tunnel: w127 -> [_ w289]
          tunnel: w174 -> [_ w286]
          tunnel: w173 -> [_ w285]
          tunnel: w104 -> [w277 w283]
          frame False {
            w282 = u32 0
            n191 = Not(x=w277) -> (.not. x?=w278:bool)
            n192 = property on="Ergebnis" class="Str"("Text.Font:Color"=w282) -> ()  [unwired: 2 in, 2 out]
            n193 = property on="Fahrzeugdaten" class="Str"("Text.Font:Color"=w282) -> ()  [unwired: 2 in, 2 out]
            n194 = property on="XY-Graph" class="XYGraph (strikt)"("Active Plot"=0, "Plot.Visible?"=TRUE ("Plot.Sichtbar"), "Active Plot"=1, "Plot.Visible?"=w278) -> ()  [unwired: 2 in, 2 out]
          }
          frame True {
            w284 = 0
            n195 = for {
              N: w289 -> [_]
              shift-right: [w311] -> w287
              shift-left: u32[] [] -> [w310]
              tunnel: w283 -> [w303]
              i -> [w305]
              w308 = 2 ("y")
              n196 = Quotient & Remainder(x=w305, y=w308) -> (x-y*floor(x/y)=w304:i32)  [unwired: 1 out]
              n197 = Equal To 0?(x=w304) -> (x = 0?=w309:bool)
              n198 = Not Equal To 0?(x=w304) -> (x != 0?=w302:bool)
              n199 = Not(x=w303) -> (.not. x?=w301:bool)
              n200 = Equal To 0?(x=w304) -> (x = 0?=w299:bool)
              n201 = And(x=w302, y=w301) -> (x .and. y?=w300:bool)
              n202 = Or(x=w299, y=w300) -> (x .or. y?=w298:bool)
              n203 = Select(t=w304, s=w299, f=w308) -> (s? t:f=w306:i32)
              n204 = property on="XY-Graph" class="XYGraph (strikt)"("Active Plot"=w305, "Plot.Visible?"=w298, "Plot.YScaleIdx"=w304, "Plot.Line Style"=w306) -> ("Plot.Plot Color"=w307:u32)  [unwired: 2 in, 2 out]
              n205 = case shown="True" w309 {
                tunnel: w307 -> [_ w315]
                tunnel: [w312 w314] -> w311
                tunnel: w310 -> [w312 w313]
                frame False {
                }
                frame True {
                  n206 = Insert Into Array(array=w313, new element=w315) -> (w314:u32[])  [unwired: 1 in]
                }
              }
            }
            n207 = for {
              shift-right: [w297] -> _
              shift-left: w284 -> [w294]
              tunnel: w287 -> [w295] mode=indexing
              tunnel: w286 -> [w296]
              tunnel: w285 -> [w293]
              shift-right: [w292] -> _
              shift-left: w284 -> [w291]
              w290 = "\t"
              n208 = Match Pattern(string=w293, regular expression=w290, offset (0)=w291) -> (offset past match=w292:i32)  [unwired: 3 out]
              n209 = Match Pattern(string=w296, regular expression=w290, offset (0)=w294) -> (offset past match=w297:i32)  [unwired: 3 out]
              n210 = property on="Fahrzeugdaten" class="Str"("Text.Selection Start"=w291, "Text.Selection End"=w292, "Text.FontColor"=w295) -> ()  [unwired: 2 in, 2 out]
              n211 = property on="Ergebnis" class="Str"("Text.Selection Start"=w294, "Text.Selection End"=w297, "Text.FontColor"=w295) -> ()  [unwired: 2 in, 2 out]
            }
          }
        }
        n212 = Max & Min(x=w127, y=2) -> (max(x,y)=w128:i32)  [unwired: 1 out]
        n213 = Greater Or Equal?(x=w127, y=14) -> (x >= y?=w159:bool)
        n214 = property on="XY-Graph" class="XYGraph (strikt)"("LegNumRows"=w128) -> ()  [unwired: 2 in, 2 out]
        n215 = case shown="True" w159 {
          frame False {
          }
          frame True {
            n216 = property on="Überlagern" class="Bool. (strikt)"("DisabledEnum"=2) -> ()  [unwired: 2 in, 2 out]
          }
        }
        "Ergebnis" <- w174
        "Fahrzeugdaten" <- w173
      }
      event "Speichern": Value Change {
        n217 = event-data() -> ("OldVal"=w365:bool)  [unwired: 1 in, 5 out]
        n218 = local write "Speichern"(w365) -> ()
        n219 = control-ref of="Datenspeicher"() -> (w364:refnum<vi>)
        n220 = call "savecluster_V0.01.vi"("Datenspeicher 2"=w364) -> ()  [unwired: 2 in]
      }
      event "Stopp": Value Change {
        n221 = event-data() -> ("OldVal"=w366:bool, "NewVal"=w367:bool)  [unwired: 1 in, 4 out]
        n222 = local write "Stopp"(w366) -> ()
      }
      event "Legende": Value Change {
        n223 = event-data() -> ()  [unwired: 1 in, 6 out]
        n224 = local read "XY-Graph"() -> (w371:cluster{dbl[], dbl[]}[])
        n225 = Array Size(array=w371) -> (size(s)=w370:i32)
        n226 = Max & Min(x=w370, y=2) -> (max(x,y)=w368:i32)  [unwired: 1 out]
        n227 = property on="XY-Graph" class="XYGraph (strikt)"("Legend Visible"="Legende", "LegNumRows"=w368) -> ()  [unwired: 2 in, 2 out]
      }
    }
  }
  n228 = property on="XY-Graph" class="XYGraph (strikt)"("Legend Visible"=TRUE, "LegNumRows"=2) -> ()  [unwired: 2 in, 2 out]
  n229 = property on="Fensterbereich" class="Bereich"("Origin"=T3 {"Horizontal"=8, "Vertical"=6}) -> ()  [unwired: 2 in, 2 out]
  n230 = property on="Fensterbereich" class="Bereich"("Origin"=T3 {"Horizontal"=8, "Vertical"=6}) -> ()  [unwired: 2 in, 2 out]
  n231 = property on="Ergebnis" class="Str"("Value"=w12) -> ()  [unwired: 2 in, 2 out]
  n232 = property on="Pmax" class="Str"("Value"=w12) -> ()  [unwired: 2 in, 2 out]
  n233 = property on="Fahrzeugdaten" class="Str"("Value"=w12) -> ()  [unwired: 2 in, 2 out]
  n234 = property on="Datum, Zeit" class="Str"("Value"=w12) -> ()  [unwired: 2 in, 2 out]
  n235 = property on="Gl. Mittelwert" class="DigWert (strikt)"("DisabledEnum"=w2) -> ()  [unwired: 2 in, 2 out]
  n236 = property on="Differenzenquotient" class="DigWert (strikt)"("DisabledEnum"=w2) -> ()  [unwired: 2 in, 2 out]
  n237 = Bundle(w8, w8) -> (w6:cluster{dbl[], dbl[]})  [unwired: 1 in]
  n238 = Bundle(w8, w8) -> (w5:cluster{dbl[], dbl[]})  [unwired: 1 in]
  n239 = case shown="True" "Berechnen" {
    selector: "Berechnen" -> [_ w376]
    frame False {
    }
    frame True {
      n240 = property on="Berechnen" class="Bool. (strikt)"("Value"=w376, "DisabledEnum"=T6."Enabled" ("Deaktiviert")) -> (error out=w373:errorcluster)  [unwired: 2 in, 1 out]
      n241 = property on="Öffnen" class="Bool. (strikt)"(error in=w373, "Val(Sgnl)"=TRUE ("Wert (signalisierend)")) -> ()  [unwired: 1 in, 2 out]
    }
  }
  n242 = property on="Berechnen" class="Bool. (strikt)"("DisabledEnum"=w4) -> ()  [unwired: 2 in, 2 out]
  n243 = property on="Überlagern" class="Bool. (strikt)"("DisabledEnum"=w4) -> ()  [unwired: 2 in, 2 out]
  n244 = property on="Speichern" class="Bool. (strikt)"("DisabledEnum"=w4) -> ()  [unwired: 2 in, 2 out]
  n245 = property on="Drucken" class="Bool. (strikt)"("DisabledEnum"=w4) -> ()  [unwired: 2 in, 2 out]
  n246 = Build Array(w6, w5) -> (w7:cluster{dbl[], dbl[]}[])
  n247 = property on="XY-Graph" class="XYGraph (strikt)"("Value"=w7) -> ()  [unwired: 2 in, 2 out]
